vi "CheckMatchesWorkingTmp.vi"(11 "Last Draw":i64[](array[numeric])) -> (0 "Resulting Match":i64[][](array[numeric]), 3 "All Matches":i32[](array[numeric]), 8 "Your Suppose":i32[][](array[numeric]))   [LabVIEW 2023]
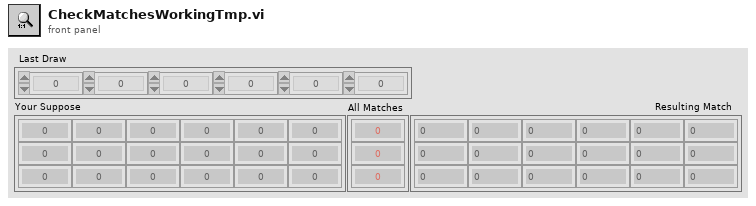
[diagram p1: front panel]
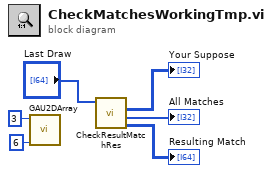
[diagram p0: block diagram]
diagram:
  n1 = call "GAU2DArray.vi"("Colums"=6, "Rows"=3) -> ()  [unwired: 8 in, 2 out]
  n2 = call "CheckResultMatchRes.vi"("Last Draw"="Last Draw") -> ("Matches array"=→"Resulting Match":i64[][], "Matches"=→"All Matches":i32[], "Your Suppose"=→"Your Suppose":i64[][])  [unwired: 7 in, 1 out]
